vi "SIM_Interval_Constructor.vi"(10 "History Data in":dbl[](array[numeric]), 11 "size(s)":i32) -> (3 "History Data out":dbl[](array[numeric]))   [LabVIEW 2022 SP3]
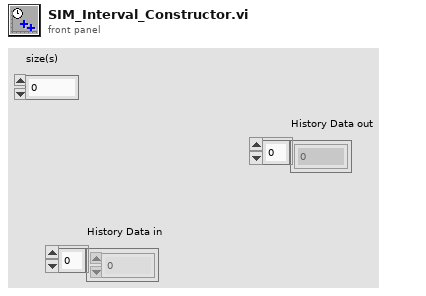
[diagram p1: front panel]
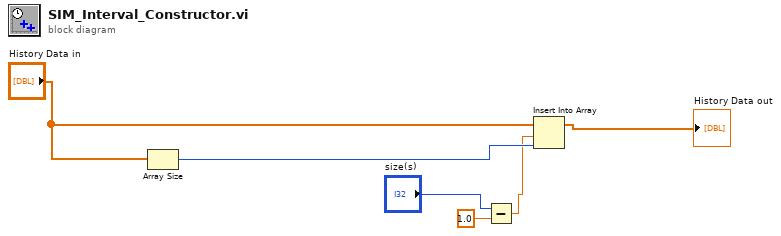
[diagram p0: block diagram]
diagram:
  n1 = Array Size(array="History Data in") -> (size(s)=w4:i32)
  n2 = Subtract(x="size(s)", y=1.0) -> (x-y=w1:dbl)
  n3 = Insert Into Array(array="History Data in", index=w1, new element=w4) -> (→"History Data out":dbl[])
